vi "Read Goto.vi"(6 "amp?":bool caption="Amps", 7 "IO Info":T1={"Address"={"Com Port"=1, "ISOBUS Address"=2, "GPIB Address"=24, "Communication"=enum."ISOBUS"}, "Version"=enum."IPS"}) -> (1 "unit":string caption="Unit", 2 "target":dbl caption="Target", 3 "display":string caption="Display")   [LabVIEW 2009, in "Magnet.lvclass"]
uses:
  Magnet.lvclass
  Oxford/PSSUBS.LLB/PSIO.ctl
  Oxford/BUSGEN.LLB/OxfordAddress.ctl
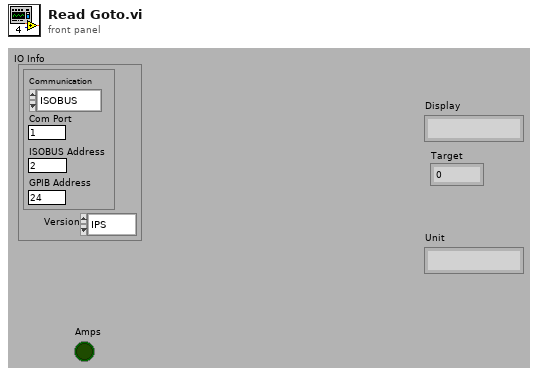
[diagram p1: front panel]
types:
  T1 = typedef "PSIO.ctl" = cluster{"Address":T2, "Version":enum16{"PS", "IPS"}}
  T2 = typedef "OxfordAddress.ctl" = cluster{"Com Port":i32, "ISOBUS Address":i32, "GPIB Address":i16, "Communication":enum16{"RS232", "ISOBUS", "GPIB", "Gateway"}}
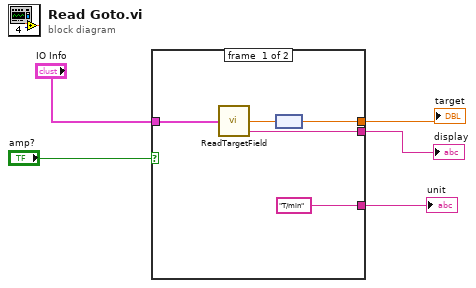
[diagram p0: block diagram]
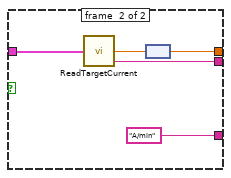
[diagram p2: hidden frame]
diagram:
  n1 = case shown="False" "amp?" {
    tunnel: "IO Info" -> [w10 w15]
    tunnel: [w8 w13] -> w2
    tunnel: [w7 w14] -> w1
    tunnel: ["T/min" "A/min"] -> w3
    frame #0 {
      n2 = call "ReadTargetField.vi"("IO Info"=w10) -> ("Target field"=w9:dbl[unit], "Display"=w7:string)  [unwired: 1 out]
      n3 = node(w9) -> (w8:dbl)
    }
    frame #1 {
      n4 = call "ReadTargetCurrent.vi"("IO Info"=w15) -> ("Target current"=w12:dbl[unit], "Display"=w14:string)  [unwired: 1 out]
      n5 = node(w12) -> (w13:dbl)
    }
  }
  "target" <- w2
  "display" <- w1
  "unit" <- w3
